vi "GetArmSource.vi"(8 "Error In":errorcluster, 11 "Keithley 6485 In":refnum<visa-resource-name>) -> (0 "Error Out":errorcluster, 2 "Arm Source":T1, 3 "Keithley 6485 Out":refnum<visa-resource-name>)   [LabVIEW 2012, in "Keithley-6485.lvlib"]
uses:
  Keithley-6485.lvlib
  Controls/ArmSource.ctl
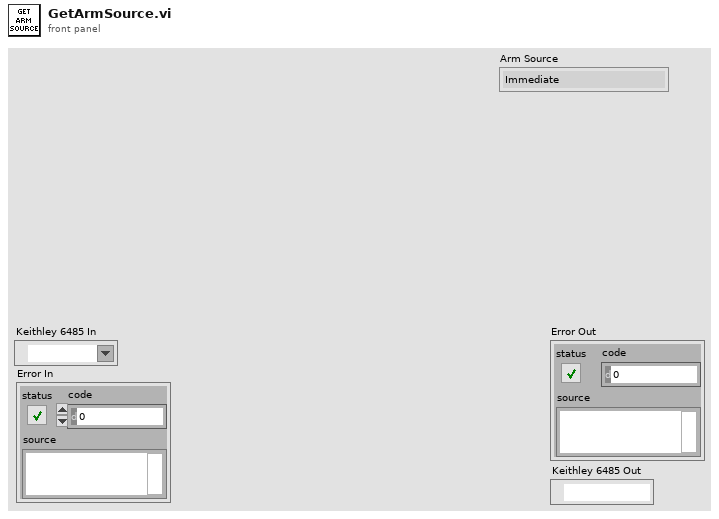
[diagram p1: front panel]
types:
  T1 = typedef "Keithley-6485.lvlib/ArmSource.ctl" = enum16{"Immediate", "Timer", "Manual", "Bus", "TLink"}
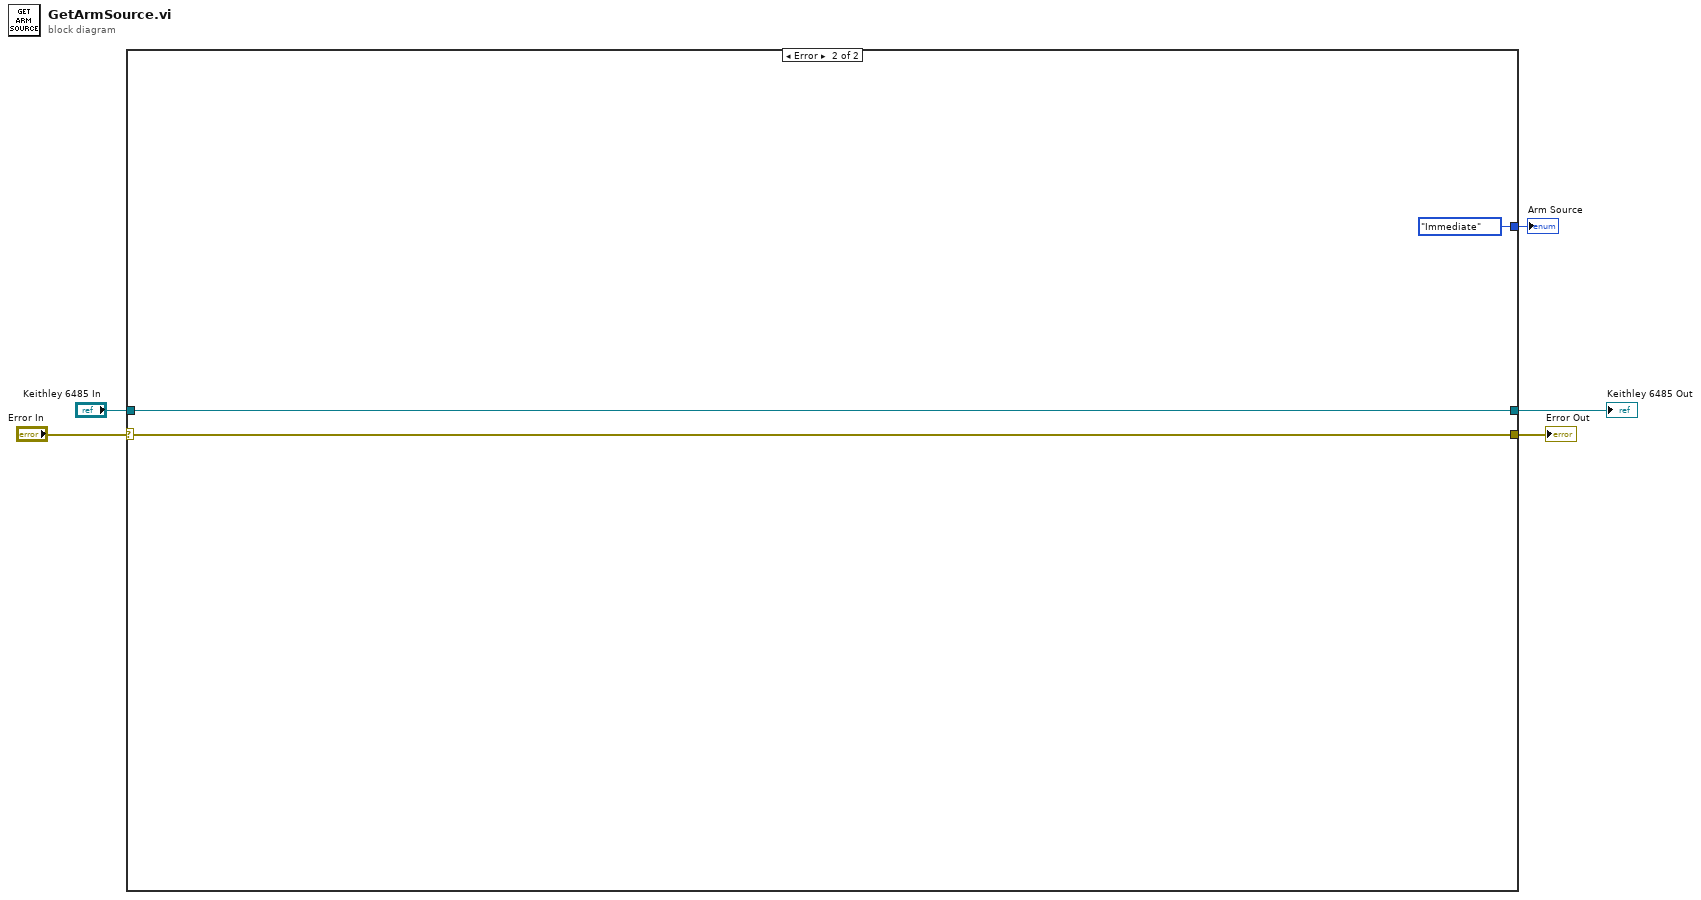
[diagram p0: block diagram]
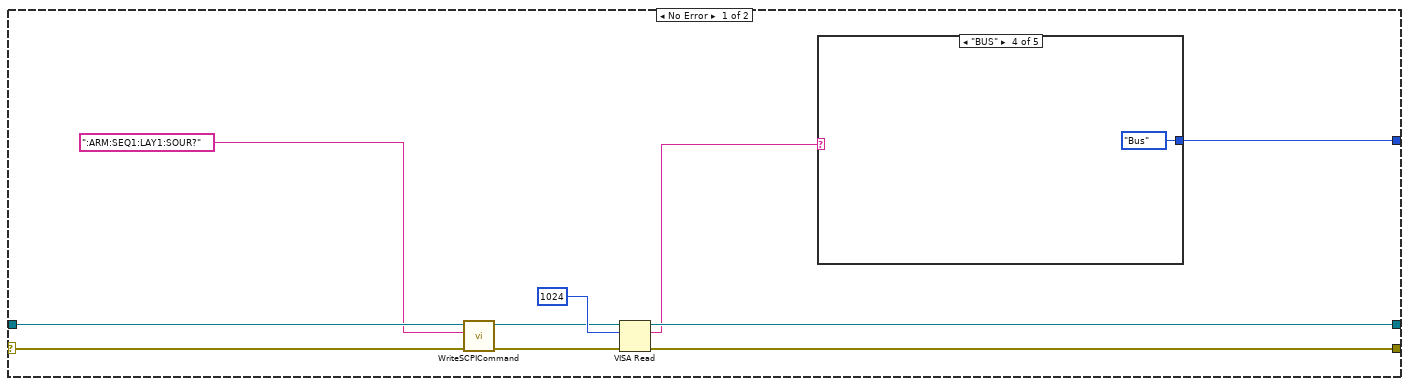
[diagram p2: hidden frame]
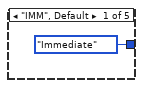
[diagram p3: hidden frame]
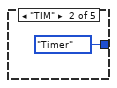
[diagram p4: hidden frame]
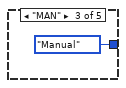
[diagram p5: hidden frame]
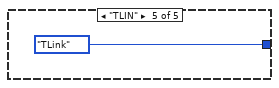
[diagram p6: hidden frame]
diagram:
  n1 = case shown="Error" "Error In" {
    selector: "Error In" -> [w10 w22]
    tunnel: "Keithley 6485 In" -> [w9 w23]
    tunnel: [w15 w22] -> w3
    tunnel: [w14 w23] -> w2
    tunnel: [w6 ArmSource."Immediate" ("Arm Source")] -> w1
    frame No Error {
      n2 = call "WriteSCPICommand.vi"("Error In"=w10, "SCPI Command"=":ARM:SEQ1:LAY1:SOUR?" ("string"), "Keithley 6482 In"=w9) -> ("Error Out"=w11:errorcluster, "Keithley 6482 Out"=w12:refnum<visa-resource-name>)  [unwired: 7 in]
      n3 = VISA Read(VISA resource name=w12, byte count=u32 1024, error in (no error)=w11) -> (VISA resource name out=w14:refnum<visa-resource-name>, read buffer=w7:string, error out=w15:errorcluster)  [unwired: 1 out]
      n4 = case shown="\"BUS\"" w7 {
        tunnel: [ArmSource."Immediate" ("Arm Source") ArmSource."Timer" ("Arm Source") ArmSource."Manual" ("Arm Source") ArmSource."Bus" ("Arm Source") ArmSource."TLink" ("Arm Source")] -> w6
        frame "IMM", Default {
        }
        frame "TIM" {
        }
        frame "MAN" {
        }
        frame "BUS" {
        }
        frame "TLIN" {
        }
      }
    }
    frame Error {
    }
  }
  "Error Out" <- w3
  "Keithley 6485 Out" <- w2
  "Arm Source" <- w1
